vi "PFI-28000-Chan-28144_Get Max Loop Resistance.vi"(8 "error in (no error)":errorcluster, 11 "PFI-28000-Chan-28144 in":refnum<class "PFI-28000-Chan-28144.lvclass">) -> (0 "error out":errorcluster, 2 "Max Loop Resistance":dbl, 3 "PFI-28000-Chan-28144 out":refnum<class "PFI-28000-Chan-28144.lvclass">)   [LabVIEW 2017, in "PFI-28000-Chan-28144.lvclass"]
uses:
  PFI-28000-Chan-28144.lvclass
  C:/wc/07143 Precision Filters 28000 Support/Driver/source/Channel/PFI-28000-Channel.lvclass
  Utilities/PFI-28000-Utils.lvlib
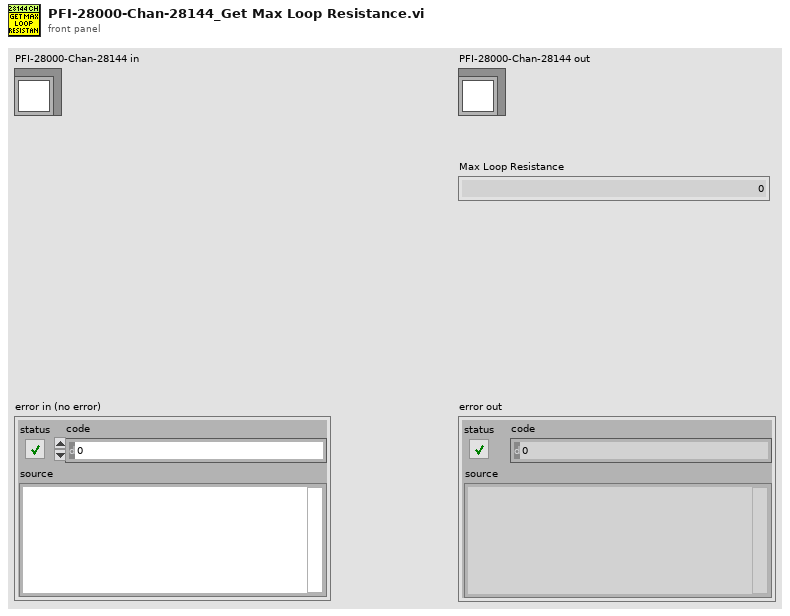
[diagram p1: front panel]
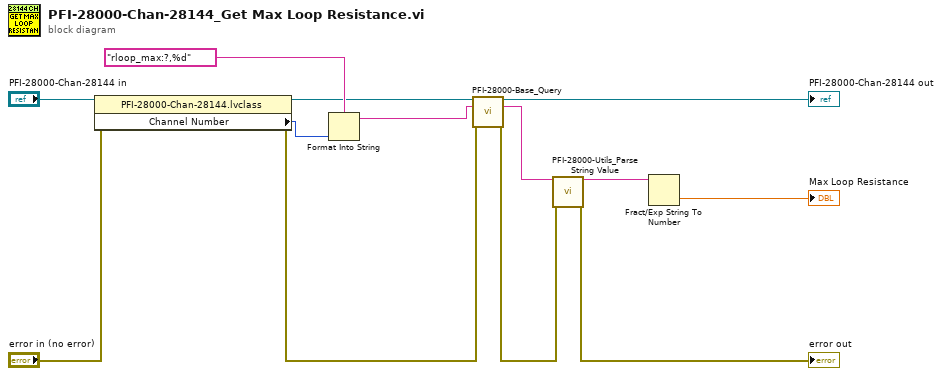
[diagram p0: block diagram]
diagram:
  n1 = property class="PFI-28000-Chan-28144.lvclass"(reference="PFI-28000-Chan-28144 in", error in="error in (no error)") -> (reference out=w7:refnum<class "PFI-28000-Chan-28144.lvclass">, error out=w9:errorcluster, "Channel Number"=w11:i32)
  n2 = Format Into String(format string="rloop_max:?,%d" ("empty string"), w11) -> (resulting string=w8:string)  [unwired: 2 in, 1 out]
  n3 = call-dynamic "PFI-28000-Base_Query.vi"("PFI-28000-Base in"=w7, "Command"=w8, "error in (no error)"=w9) -> ("PFI-28000-Base out"=→"PFI-28000-Chan-28144 out":refnum<class "PFI-28000-Chan-28144.lvclass">, "Response"=w1:string, "error out"=w3:errorcluster)  [unwired: 9 in, 1 out]
  n4 = call "PFI-28000-Utils_Parse String Value.vi"("String"=w1, "error in (no error)"=w3) -> ("String Value"=w4:string, "error out"=→"error out":errorcluster)  [unwired: 11 in, 1 out]
  n5 = Fract/Exp String To Number(string=w4) -> (number=→"Max Loop Resistance":dbl)  [unwired: 3 in, 1 out]
